vi "Protected Read (1D I8).vi"(7 "count (-1: all)":i64=-1 format="%d elements", 8 "error in (no error)":errorcluster, 9 "offset (0)":u64 format="%d bytes", 10 "buffer in":i8[](array[numeric]), 11 "Pointer in":refnum<class "Pointer.lvclass">) -> (0 "error out":errorcluster, 1 "offset out":u64 format="%d bytes", 2 "buffer out":i8[](array[numeric]), 3 "Pointer out":refnum<class "Pointer.lvclass">)   [LabVIEW 2017, in "Memory Manager.lvlib" / "Pointer.lvclass"]
doc: "Reads the contents of the address specified by <b>pointer + offset</b> into <b>value</b>.\n\n<b>Note:</b> This VI is <b>safe</b>.\n\nSafe means that this function evaluates the size parameter of <b>pointer</b> to ensure that is inbounds of allocated memory before peforming a memory read/write. Reading/writing more data to a pointer than it has allocated can corrupt or crash LabVIEW."
uses:
  Pointer.lvclass
  Read/Read (1D I8).vi
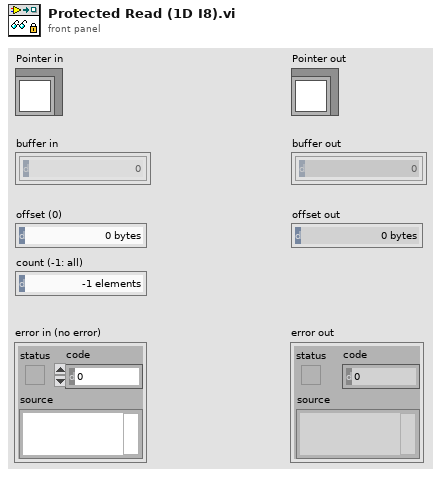
[diagram p1: front panel]
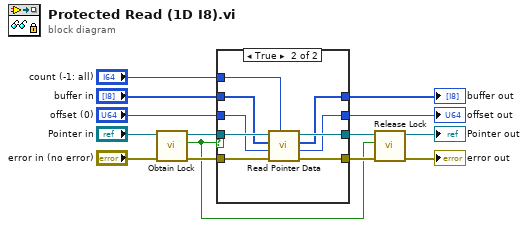
[diagram p0: block diagram]
diagram:
  n1 = call-dynamic "Obtain Lock.vi"("error in (no error)"="error in (no error)", "Pointer in"="Pointer in") -> ("error out"=w8:errorcluster, "lock status"=w2:bool, "Pointer out"=w9:refnum<class "Pointer.lvclass">)  [unwired: 6 in, 1 out]
  n2 = case shown="True" w2 {
    tunnel: [w18 w27] -> w14
    tunnel: [w15 w26] -> w13
    tunnel: [w16 w25] -> w12
    tunnel: w9 -> [w18 w24]
    tunnel: w8 -> [w17 w23]
    tunnel: "buffer in" -> [w15 w22]
    tunnel: "offset (0)" -> [w16 w21]
    tunnel: [w17 w20] -> w5
    tunnel: "count (-1: all)" -> [_ w19]
    frame False {
    }
    frame True {
      n3 = call-poly "Read Pointer Data.vi"("count (-1: all)"=w19, "error in (no error)"=w23, "offset (0)"=w21, "buffer in"=w22, "Pointer in"=w24) -> ("error out"=w20:errorcluster, "offset out"=w25:u64, "buffer out"=w26:i8[], "Pointer out"=w27:refnum<class "Pointer.lvclass">)  [unwired: 3 in]
    }
  }
  "buffer out" <- w13
  "offset out" <- w12
  n4 = call-dynamic "Release Lock.vi"("error in (no error)"=w5, "new lock status (T)"=w2, "Pointer in"=w14) -> ("error out"=→"error out":errorcluster, "Pointer out"=→"Pointer out":refnum<class "Pointer.lvclass">)  [unwired: 6 in, 1 out]
